vi "Create Plot Object.vi"(6 "Control Ref Queue":T1, 7 "Actual Transform In":T2, 8 "error in (no error)":errorcluster, 9 "Multiplot Representation In":T4, 10 "3D Contour.lvclass in":refnum<class "3D Contour.lvclass">, 11 "Plot Object In":refnum<vi>) -> (0 "error out":errorcluster, 1 "Multiplot Representation Out":T4, 2 "3D Contour.lvclass out":refnum<class "3D Contour.lvclass">, 3 "Plot Object Out":refnum<vi>, 5 "Actual Transform Out":T2)   [LabVIEW 2020, in "3D Contour.lvclass"]
uses:
  <vilib>/Math Plots/3D Math Plots/3D Contour/3D Contour/3D Contour.lvclass
  <vilib>/Math Plots/3D Math Plots/3D Plot/3D Plot/Typedef/Multiplot Representation.ctl
  <vilib>/Math Plots/3D Math Plots/3D Plot/3D Plot/Typedef/Plot Representation.ctl
  <vilib>/Math Plots/3D Math Plots/3D Plot/3D Plot/Typedef/Range Clusters.ctl
  <vilib>/Math Plots/3D Math Plots/3D Plot/3D Plot/Typedef/Mesh Data.ctl
  <vilib>/Math Plots/3D Math Plots/3D Plot/3D Plot/Typedef/Actual Transform.ctl
  <vilib>/Math Plots/3D Math Plots/3D Plot/Action String/3DMathPlot Ctrl Act Queue.ctl
  <vilib>/Math Plots/3D Math Plots/3D Plot/Action String/3DMathPlot Ctrl Act Cluster.ctl
  <vilib>/Math Plots/3D Math Plots/3D Plot/Action String/3DMathPlot State Class.ctl
  <vilib>/Math Plots/3D Math Plots/3D Contour/3D Contour/3D Contour.lvclass/3D Contour.ctl
  <vilib>/Math Plots/3D Math Plots/3D Plot/3D Plot/3D Plot.lvclass
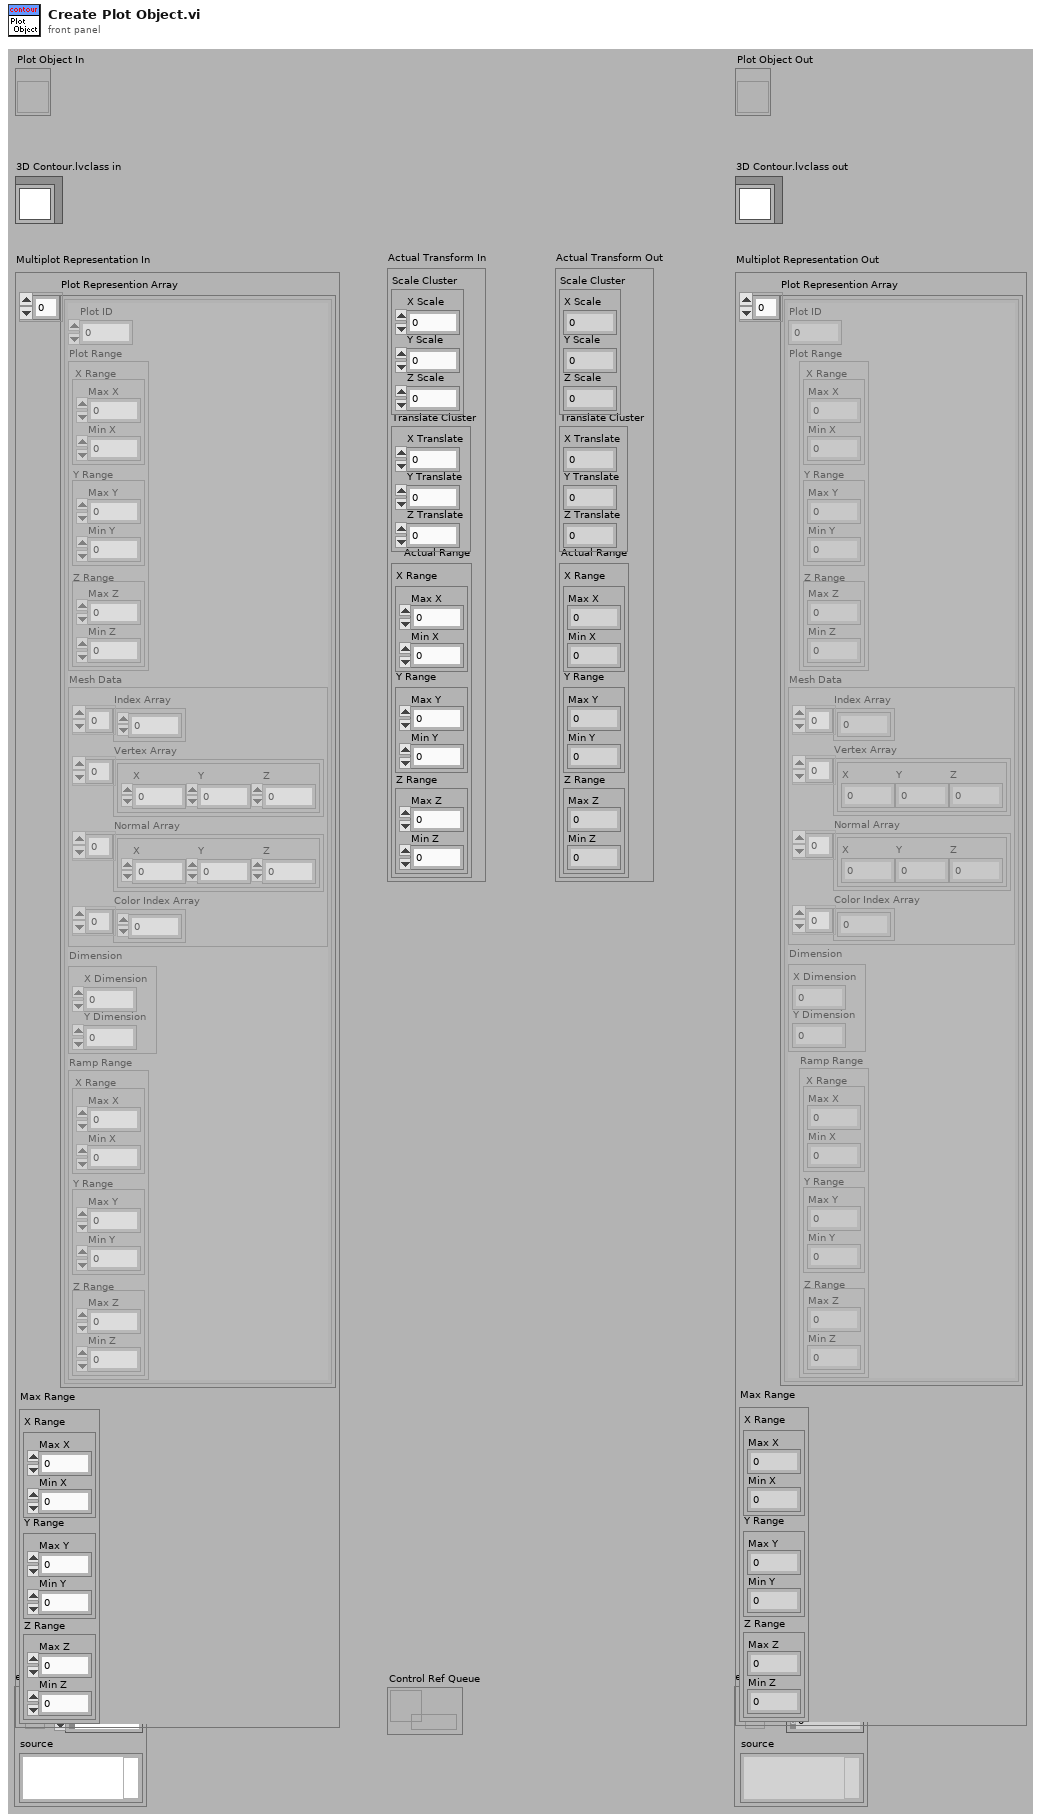
[diagram p1: front panel]
types:
  T1 = typedef "3DMathPlot Ctrl Act Queue.ctl" = refnum<queue>
  T2 = typedef "3D Plot.lvclass/Actual Transform.ctl" = cluster{"Scale Cluster":cluster{"X Scale":sgl, "Y Scale":sgl, "Z Scale":sgl}, "Translate Cluster":cluster{"X Translate":sgl, "Y Translate":sgl, "Z Translate":sgl}, "Actual Range":T3}
  T3 = typedef "3D Plot.lvclass/Range Clusters.ctl" = cluster{"X Range":cluster{"Max X":sgl, "Min X":sgl}, "Y Range":cluster{"Max Y":sgl, "Min Y":sgl}, "Z Range":cluster{"Max Z":sgl, "Min Z":sgl}}
  T4 = typedef "3D Plot.lvclass/Multiplot Representation.ctl" = cluster{"Plot Represention Array":T5[], "Max Range":T3}
  T5 = typedef "3D Plot.lvclass/Plot Representation.ctl" = cluster{"Plot ID":i32, "Plot Range":T3, "Mesh Data":T6, "Dimension":cluster{"X Dimension":i32, "Y Dimension":i32}, "Ramp Range":T3}
  T6 = typedef "3D Plot.lvclass/Mesh Data.ctl" = cluster{"Index Array":u32[], "Vertex Array":cluster{"X":sgl, "Y":sgl, "Z":sgl}[], "Normal Array":cluster{"X":sgl, "Y":sgl, "Z":sgl}[], "Color Index Array":i32[]}
  T7 = typedef "3D Contour.lvclass/3D Contour Property Array.ctl" = T8[]
  T8 = typedef "3D Contour.lvclass/3D Contour Property.ctl" = cluster{"General Property":cluster{"Plot Name":string, "Coordinate System":enum16{"Cartesian", "Cylindrical", "Spherical"}, "Opacity":sgl}, "Projection Property":cluster{"Draw XY":bool, "Draw YZ":bool, "Draw XZ":bool}, "Plot Property":cluster{"Line Style":T9, "Line Width":sgl, "Line Color":u32, "Antialiasing":bool, "Color Ramp Cluster":T10}, "Contour Property":cluster{"Contour Type":enum16{"Contour", "Contour with surface"}, "Axis Basis":enum16{"X-Axis", "Y-Axis", "Z-Axis"}, "Level List":sgl[], "Level Mode":enum16{"Levels", "Interval", "Level List"}, "Levels":u16, "Interval":sgl}}
  T9 = typedef "3D Plot.lvclass/Line Type.ctl" = enum16{"None", "Solid", "Dash", "Dot", "Dash Dot"}
  T10 = typedef "3D Plot.lvclass/Color Ramp Cluster.ctl" = cluster{"Color Ramp Style":enum16{"None", "Shaded", "Color spectrum", "Grey scale", "Custom"}, "Color Ramp Array":u32[], "Color Ramp Index":i32[], "Interpolate?":bool, "Logarithm?":bool}
  T11 = enum16{"Points", "Lines", "Line Strip", "Line Loop", "Triangles", "Triangle Strip", "Triangle Fan", "Quads", "Quad Strip", "Polygon"}
  T12 = cluster{"Draw XY":bool, "Draw YZ":bool, "Draw XZ":bool}
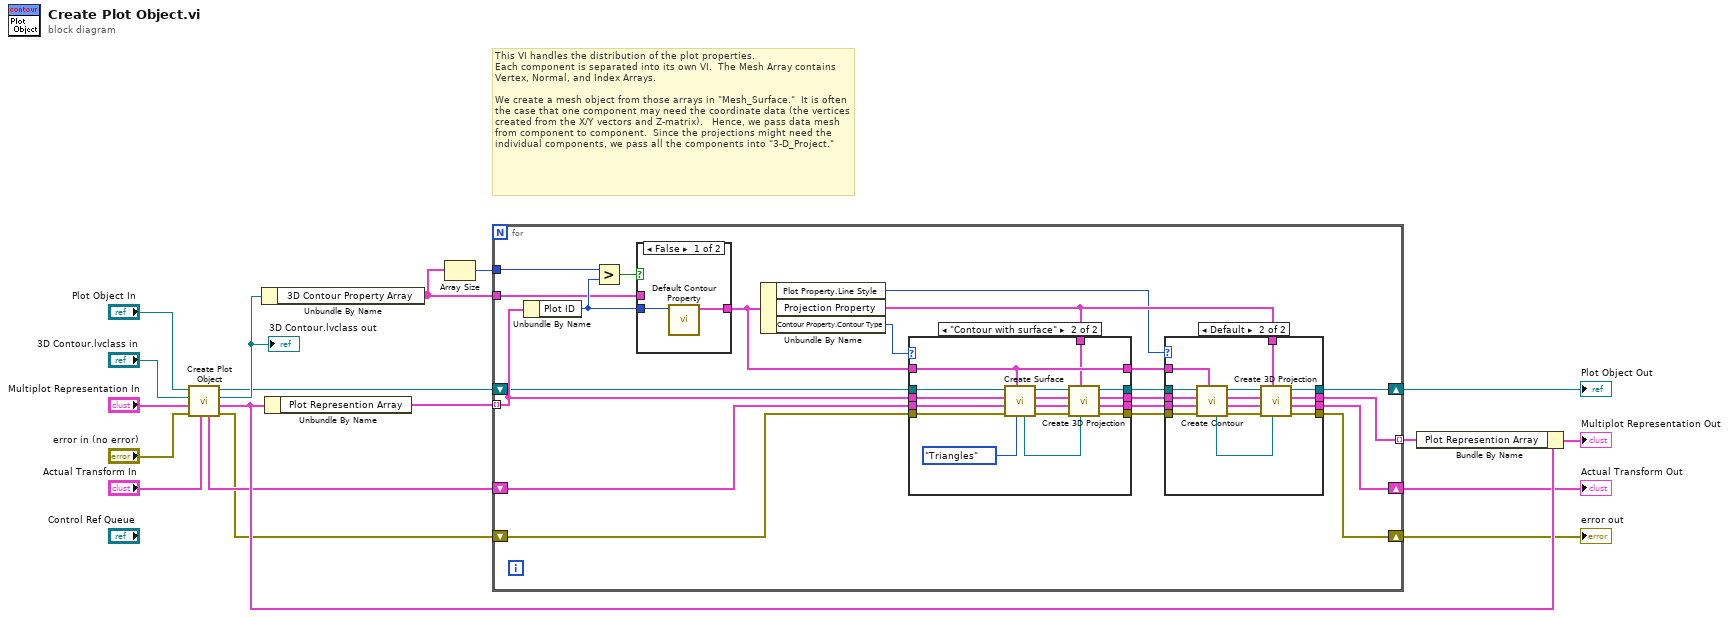
[diagram p0: block diagram]
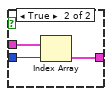
[diagram p2: hidden frame]
diagram:
  # "This VI handles the distribution of the plot properties.  \nEach component is separated into its own VI.  The Mesh Array contains Vertex, Normal, and Index Arrays.  \n\nWe create a mesh object from those arrays in \"Mesh_Surface.\"  It is often the case that one component may need the coordinate data (the vertices created from the X/Y vectors and Z-matrix).   Hence, we pass data mesh from component to component.  Since the projections might need the individual components, we pass all the components into \"3-D_Project.\""
  n1 = call-parent "Create Plot Object.vi"("Actual Transform In"="Actual Transform In", "error in (no error)"="error in (no error)", "Multiplot Representation In"="Multiplot Representation In", "3D Plot.lvclass in"="3D Contour.lvclass in", "Plot Object In"="Plot Object In") -> ("error out"=w5:errorcluster, "Multiplot Representation Out"=w13:T4, "3D Plot.lvclass out"=w6:refnum<class "3D Contour.lvclass">, "Plot Object Out"=w4:refnum<vi>, "Actual Transform Out"=w9:T2)  [unwired: 2 in]
  "3D Contour.lvclass out" <- w6
  n2 = Unbundle By Name(w6) -> ("3D Contour Property Array"=w2:T7)
  n3 = Unbundle By Name(w13) -> ("Plot Represention Array"=w18:T5[])
  n4 = Array Size(array=w2) -> (size(s)=w1:i32)
  n5 = for {
    tunnel: [w38] -> w17 mode=indexing
    tunnel: w2 -> [w20]
    shift-right: [w39] -> w3
    shift-left: w4 -> [w32]
    shift-right: [w36] -> w7
    shift-left: w5 -> [w35]
    shift-right: [w37] -> w8
    shift-left: w9 -> [w34]
    tunnel: w18 -> [w33] mode=indexing
    tunnel: w1 -> [w19]
    n6 = Unbundle By Name(w33) -> ("Plot ID"=w22:i32)
    n7 = Greater?(x=w19, y=w22) -> (0:w23:bool)
    n8 = case shown="False" w23 {
      tunnel: w20 -> [_ w44]
      tunnel: [w40 w43] -> w21
      tunnel: w22 -> [w41 w42]
      frame False {
        n9 = call <vilib>:"Default Contour Property.vi"("Plot ID"=w41) -> ("Default Property"=w40:T8)  [unwired: 10 out]
      }
      frame True {
        n10 = Index Array(array=w44, index=w42) -> (element=w43:T8)
      }
    }
    n11 = Unbundle By Name(w21) -> ("Plot Property.Line Style"=w24:T9, "Projection Property"=w25:T12, "Contour Property.Contour Type"=w26:enum16{"Contour", "Contour with surface"})
    n12 = case shown="\"Contour with surface\"" w26 {
      tunnel: w25 -> [_ w68]
      tunnel: w32 -> [w67 w78]
      tunnel: w33 -> [w66 w77]
      tunnel: w34 -> [w65 w76]
      tunnel: w35 -> [w64 w75]
      tunnel: [w67 w74] -> w31
      tunnel: [w66 w73] -> w30
      tunnel: [w65 w72] -> w29
      tunnel: [w64 w71] -> w28
      tunnel: w21 -> [w63 w69]
      tunnel: [w63 w69] -> w27
      frame "Contour", Default {
      }
      frame "Contour with surface" {
        n13 = call <vilib>:"Create Surface.vi"("Draw Mode"=T11."Triangles", "3D Contour Property"=w69, "error in (no error)"=w75, "Actual Transform In"=w76, "Plot Representation In"=w77, "Plot Object In"=w78) -> ("error out"=w80:errorcluster, "Actual Transform Out"=w81:T2, "Plot Representation Out"=w73:T5, "Plot Object Out"=w82:refnum<vi>, "Surface Object Out"=w79:refnum<vi>)  [unwired: 1 in]
        n14 = call <vilib>:"Create 3D Projection.vi"("Sub Object In"=w79, "Projection Property"=w68, "error in (no error)"=w80, "Actual Transform In"=w81, "Plot Object In"=w82) -> ("error out"=w71:errorcluster, "Actual Transform Out"=w72:T2, "Plot Object Out"=w74:refnum<vi>)  [unwired: 1 in, 3 out]
      }
    }
    n15 = case shown="Default" w24 {
      tunnel: [w48 w58] -> w39
      tunnel: [w47 w57] -> w38
      tunnel: [w46 w56] -> w37
      tunnel: [w45 w55] -> w36
      tunnel: w25 -> [_ w54]
      tunnel: w31 -> [w48 w53]
      tunnel: w30 -> [w47 w52]
      tunnel: w29 -> [w46 w51]
      tunnel: w28 -> [w45 w50]
      tunnel: w27 -> [_ w49]
      frame "None" {
      }
      frame Default {
        n16 = call <vilib>:"Create Contour.vi"("3D Contour Property"=w49, "error in (no error)"=w50, "Actual Transform In"=w51, "Plot Representation In"=w52, "Plot Object In"=w53) -> ("error out"=w62:errorcluster, "Actual Transform Out"=w60:T2, "Plot Representation Out"=w57:T5, "Plot Object Out"=w61:refnum<vi>, "Contour Object Out"=w59:refnum<vi>)  [unwired: 2 in]
        n17 = call <vilib>:"Create 3D Projection.vi"("Sub Object In"=w59, "Projection Property"=w54, "error in (no error)"=w62, "Actual Transform In"=w60, "Plot Object In"=w61) -> ("error out"=w55:errorcluster, "Actual Transform Out"=w56:T2, "Plot Object Out"=w58:refnum<vi>)  [unwired: 1 in, 3 out]
      }
    }
  }
  "error out" <- w7
  "Plot Object Out" <- w3
  "Actual Transform Out" <- w8
  n18 = Bundle By Name(cluster=w13, "Plot Represention Array"=w17) -> (→"Multiplot Representation Out":T4)
